vi "Filter and Remove Tabs and Spaces.vi"(1 "Input String":string) -> (0 "Filtered String":string)   [LabVIEW 2021]
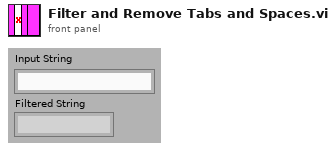
[diagram p1: front panel]
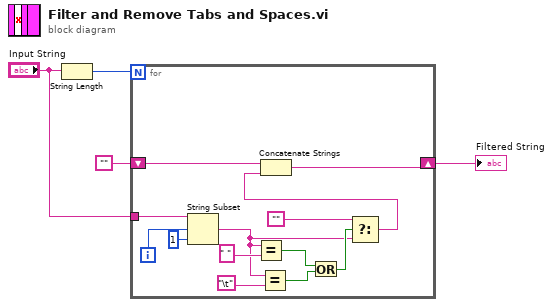
[diagram p0: block diagram]
diagram:
  n1 = String Length(string="Input String") -> (length=w4:i32)
  n2 = for {
    N: w4 -> [_]
    shift-right: [w12] -> w1
    shift-left: "" -> [w17]
    tunnel: "Input String" -> [w16]
    i -> [w15]
    n3 = String Subset(string=w16, offset (0)=w15, length (rest)=1 ("length (rest)")) -> (substring=w7:string)
    n4 = Equal?(x=w7, y=" ") -> (x = y?=w8:bool)
    n5 = Equal?(x=w7, y="\t") -> (x = y?=w5:bool)
    n6 = Or(x=w8, y=w5) -> (x .or. y?=w9:bool)
    n7 = Select(t="", s=w9, f=w7) -> (s? t:f=w13:string)
    n8 = Concatenate Strings(w17, w13) -> (w12:string)
  }
  "Filtered String" <- w1
